vi "Write Tester Rx.vi"(8 "error in (no error)":errorcluster, 11 "Panel in":refnum<class "Station Actor.lvclass">) -> (0 "error out":errorcluster, 3 "Panel out":refnum<class "Station Actor.lvclass">)   [LabVIEW 2019, in "Station Actor.lvlib" / "Station Actor.lvclass"]
uses:
  Station Actor.lvclass
  Station Actor.lvclass/Station Actor.ctl
  <vilib>/OPCUA/server/Write Variant.vi
  <vilib>/OPCUA/NI OPC UA Server.lvlib
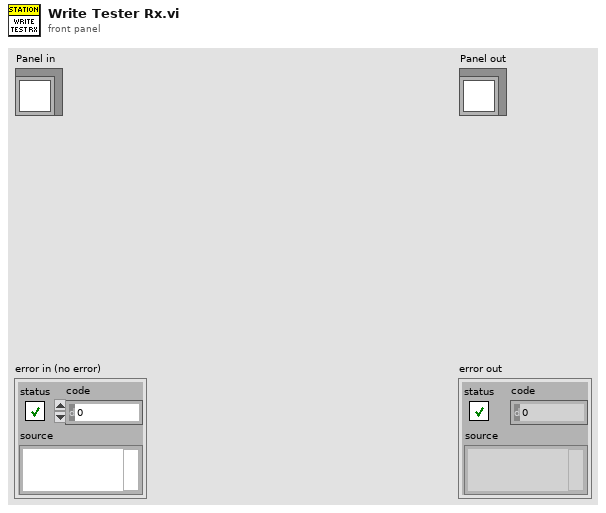
[diagram p1: front panel]
types:
  T1 = typedef "OPC UA Server Refnum.ctl" = refnum<k21>
  T2 = typedef "NodeId.ctl" = string
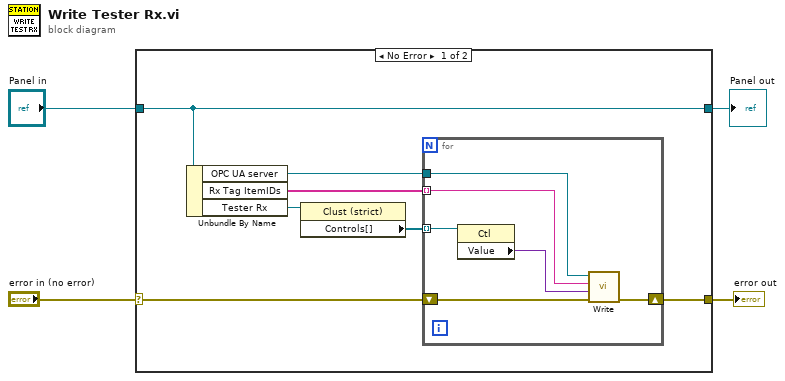
[diagram p0: block diagram]
diagram:
  n1 = case shown="No Error" "error in (no error)" {
    selector: "error in (no error)" -> [w7 w19]
    tunnel: [w6 w19] -> w3
    tunnel: [w11 w18] -> w1
    tunnel: "Panel in" -> [w11 w18]
    frame No Error {
      n2 = Unbundle By Name(w11) -> ("OPC UA server"=w9:T1, "Rx Tag ItemIDs"=w8:T2[], "Tester Rx"=w5:refnum<vi>)
      n3 = property class="Clust (strict)"(reference=w5) -> ("Controls[]"=w10:refnum<vi>[])  [unwired: 1 in, 2 out]
      n4 = for {
        tunnel: w9 -> [w17]
        tunnel: w8 -> [w15] mode=indexing
        tunnel: w10 -> [w14] mode=indexing
        shift-right: [w16] -> w6
        shift-left: w7 -> [w12]
        n5 = property class="Ctl"(reference=w14) -> ("Value"=w13:variant)  [unwired: 1 in, 2 out]
        n6 = call-poly <vilib>:"Write.vi"("error in (no error)"=w12, "value"=w13, "node ID"=w15, "OPC UA server refnum in"=w17) -> ("error out"=w16:errorcluster)  [unwired: 5 in, 2 out]
      }
    }
    frame Error {
    }
  }
  "error out" <- w3
  "Panel out" <- w1
